vi "write_attributes.vi"(8 "error in (no error)":errorcluster, 10 "attributes":T1, 11 "AdaBoostRegressor in":refnum<class "AdaBoostRegressor.lvclass">) -> (0 "error out":errorcluster, 3 "AdaBoostRegressor out":refnum<class "AdaBoostRegressor.lvclass">)   [LabVIEW 2020, in "AdaBoostRegressor.lvclass"]
uses:
  AdaBoostRegressor.lvclass
  Controls/adaboostregressor_attributes.ctl
  AdaBoostRegressor.lvclass/AdaBoostRegressor.ctl
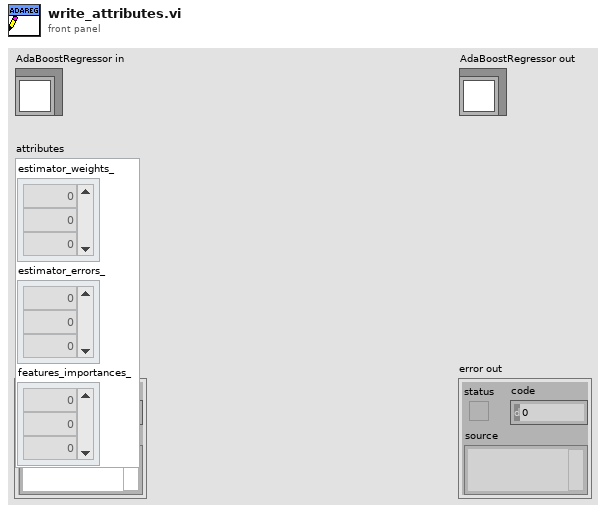
[diagram p1: front panel]
types:
  T1 = typedef "adaboostregressor_attributes.ctl" = cluster{"estimator_weights_":dbl[], "estimator_errors_":dbl[], "features_importances_":dbl[]}
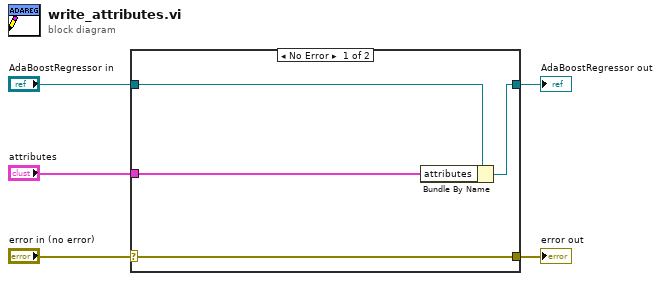
[diagram p0: block diagram]
diagram:
  n1 = case shown="No Error" "error in (no error)" {
    selector: "error in (no error)" -> [w9 w10]
    tunnel: [w9 w10] -> w4
    tunnel: [w7 w11] -> w2
    tunnel: "AdaBoostRegressor in" -> [w8 w11]
    tunnel: "attributes" -> [w6 _]
    frame No Error {
      n2 = Bundle By Name(cluster=w8, "attributes"=w6) -> (w7:refnum<class "AdaBoostRegressor.lvclass">)
    }
    frame Error {
    }
  }
  "error out" <- w4
  "AdaBoostRegressor out" <- w2
